vi "Read configuration.vi"(8 "error in (no error)":errorcluster, 11 "DIO Instrument in":refnum<class "Digital IO Instrument.lvclass">) -> (0 "error out":errorcluster, 2 "configuration":refnum<class "CEF_serializable configuration.lvclass">, 3 "DIO Instrument out":refnum<class "Digital IO Instrument.lvclass">)   [LabVIEW 2025, in "Digital IO.lvlib" / "Digital IO Instrument.lvclass"]
uses:
  Digital IO Instrument.lvclass
  Users/Public/Documents/Sandia National Labs/TSS Plugin/CEF.lvlibp/serializable configuration/CEF_serializable configuration.lvclass
  Digital IO Instrument.lvclass/Digital IO Instrument.ctl
  Users/Public/Documents/Sandia National Labs/TSS Plugin/Abstract Engine.lvlibp/Plugin/Abstract/Instrument configuration/Instrument configuration.lvclass
  C:/Users/Public/Documents/Sandia National Labs/TSS Plugin/CEF.lvlibp/serializable configuration/CEF_serializable configuration.lvclass
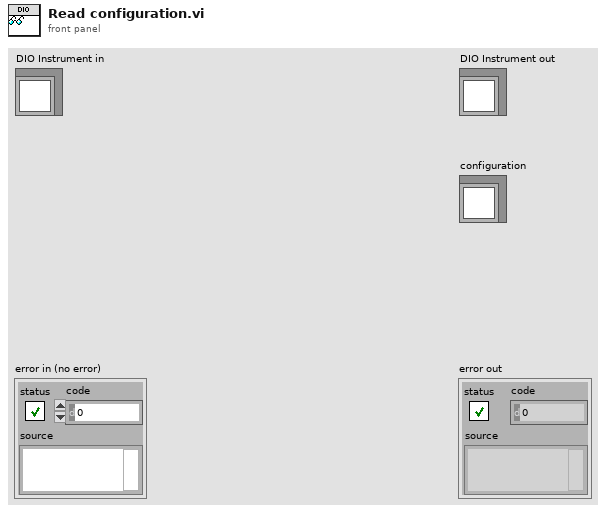
[diagram p1: front panel]
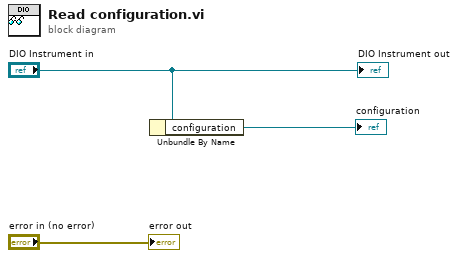
[diagram p0: block diagram]
diagram:
  n1 = Unbundle By Name("DIO Instrument in") -> ("configuration"=→"configuration":refnum<class "Instrument configuration.lvclass">)
  "error out" <- "error in (no error)"
  "DIO Instrument out" <- "DIO Instrument in"
